vi "Write rioHandler.vi"(8 "error in (no error)":errorcluster, 10 "rioHandler":refnum<class "IRIOHandler.lvclass">, 11 "CompactRIO in":refnum<class "CompactRIO.lvclass">) -> (0 "error out":errorcluster, 3 "CompactRIO out":refnum<class "CompactRIO.lvclass">)   [LabVIEW 2012, in "CompactRIO.lvclass"]
uses:
  CompactRIO.lvclass
  C/Program Files (x86)/National Instruments/LabVIEW 2012/user.lib/Common/ComponentModel/ComponentModelRT/RIOHandler/IRIOHandler/IRIOHandler.lvclass
  CompactRIO.lvclass/CompactRIO.ctl
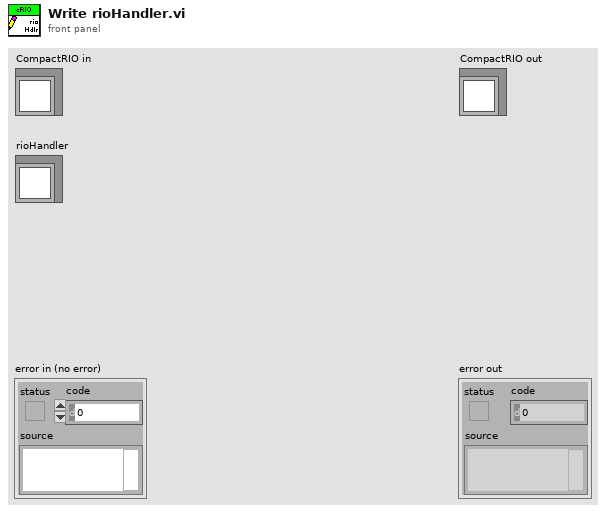
[diagram p1: front panel]
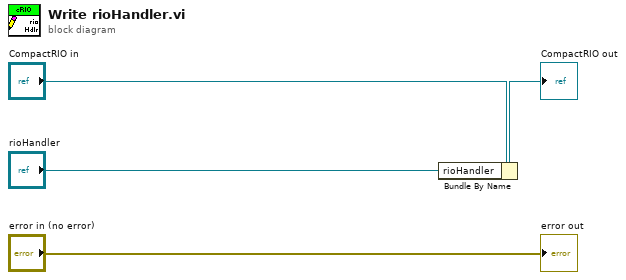
[diagram p0: block diagram]
diagram:
  n1 = Bundle By Name(cluster="CompactRIO in", "rioHandler"="rioHandler") -> (→"CompactRIO out":refnum<class "CompactRIO.lvclass">)
  "error out" <- "error in (no error)"
